vi "Create Group Buffers.vi"(8 "error in (no error)":errorcluster, 10 "Framework Configuration":refnum<class "Framework Configuration.lvclass">, 11 "VeriStand DSF in":refnum<class "VeriStand DSF.lvclass">) -> (0 "error out":errorcluster, 2 "Group Buffers":refnum<class "Buffers.lvclass">[](array[class]), 3 "VeriStand DSF out":refnum<class "VeriStand DSF.lvclass">)   [LabVIEW 2017, in "DSF Engine.lvlib" / "VeriStand DSF.lvclass"]
uses:
  VeriStand DSF.lvclass
  DSF Core.lvlibp/Classes/Buffers/Buffers.lvclass
  DSF Core.lvlibp/Classes/Configuration/Core/Framework/Framework Configuration.lvclass
  VeriStand DSF.lvclass/VeriStand DSF.ctl
  <vilib>/NI Veristand/Custom Device API/Data Access Type.ctl
  DSF Core.lvlibp/Typedefs/DSF Direction.ctl
  Shared/Data Channel Page GUID.vi
  DSF Core.lvlibp/Classes/Configuration/Core/Group/Group Configuration.lvclass
  Shared/DSF Shared.lvlib
  <vilib>/NI Veristand/Custom Device API/Custom Device API.lvlib
  DSF Core.lvlibp
  DSF Core.lvlibp/Classes/Configuration/Core/Transfer/Transfer Configuration.lvclass
  DSF Core.lvlibp/Classes/Configuration/Core/Thread/Thread Configuration.lvclass
  DSF Core.lvlibp/Classes/Configuration/Core/Plugin/Plugin Configuration.lvclass
  DSF Core.lvlibp/Classes/Buffer/Buffer.lvclass
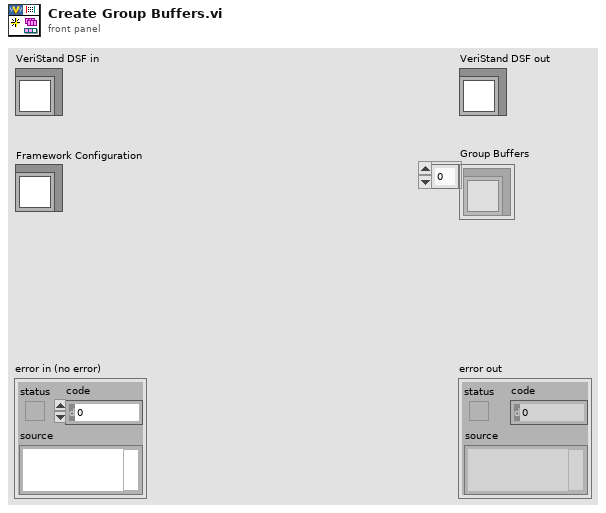
[diagram p1: front panel]
types:
  T1 = typedef "Custom Device API.lvlib/Custom Device Item Ref.ctl" = u64
  T2 = typedef "Custom Device API.lvlib/Data Access Type.ctl" = enum16{"Read", "Write"}
  T3 = typedef "DSF Core.lvlibp/DSF Direction.ctl" = enum8{"Tx", "Rx"}
  T4 = typedef "DSF Core.lvlibp/Group Configuration.lvclass/Core Group Configuration.ctl" = cluster{"name":string, "direction":T3, "cycle timing":T5, "timeout behavior":T6, "enable conversion":bool}
  T5 = typedef "DSF Core.lvlibp/DSF Timing Info.ctl" = cluster{"priority":u64, "decimation":u64, "offset":u64}
  T6 = typedef "DSF Core.lvlibp/DSF Timeout Behavior.ctl" = enum8{"Increment Late Count", "Throw Error"}
  T7 = typedef "DSF Core.lvlibp/Transfer Configuration.lvclass/Channel Configuration.ctl" = cluster{"configuration":T8, "component settings":T10[]}
  T8 = typedef "DSF Core.lvlibp/Channel Configuration.lvclass/Core Channel Configuration.ctl" = cluster{"name":string, "units":string, "engine data type":T9, "string data type":T9, "string offset":u64}
  T9 = typedef "DSF Core.lvlibp/DSF Data Type.ctl" = enum8{"Bool", "SGL", "DBL", "I8", "I16", "I32", "I64", "U8", "U16", "U32", "U64"}
  T10 = typedef "DSF Core.lvlibp/DSF Settings Info.ctl" = cluster{"component":string, "values":cluster{"key":string, "value":string}[]}
  T11 = typedef "Custom Device API.lvlib/Data Reference.ctl" = i32
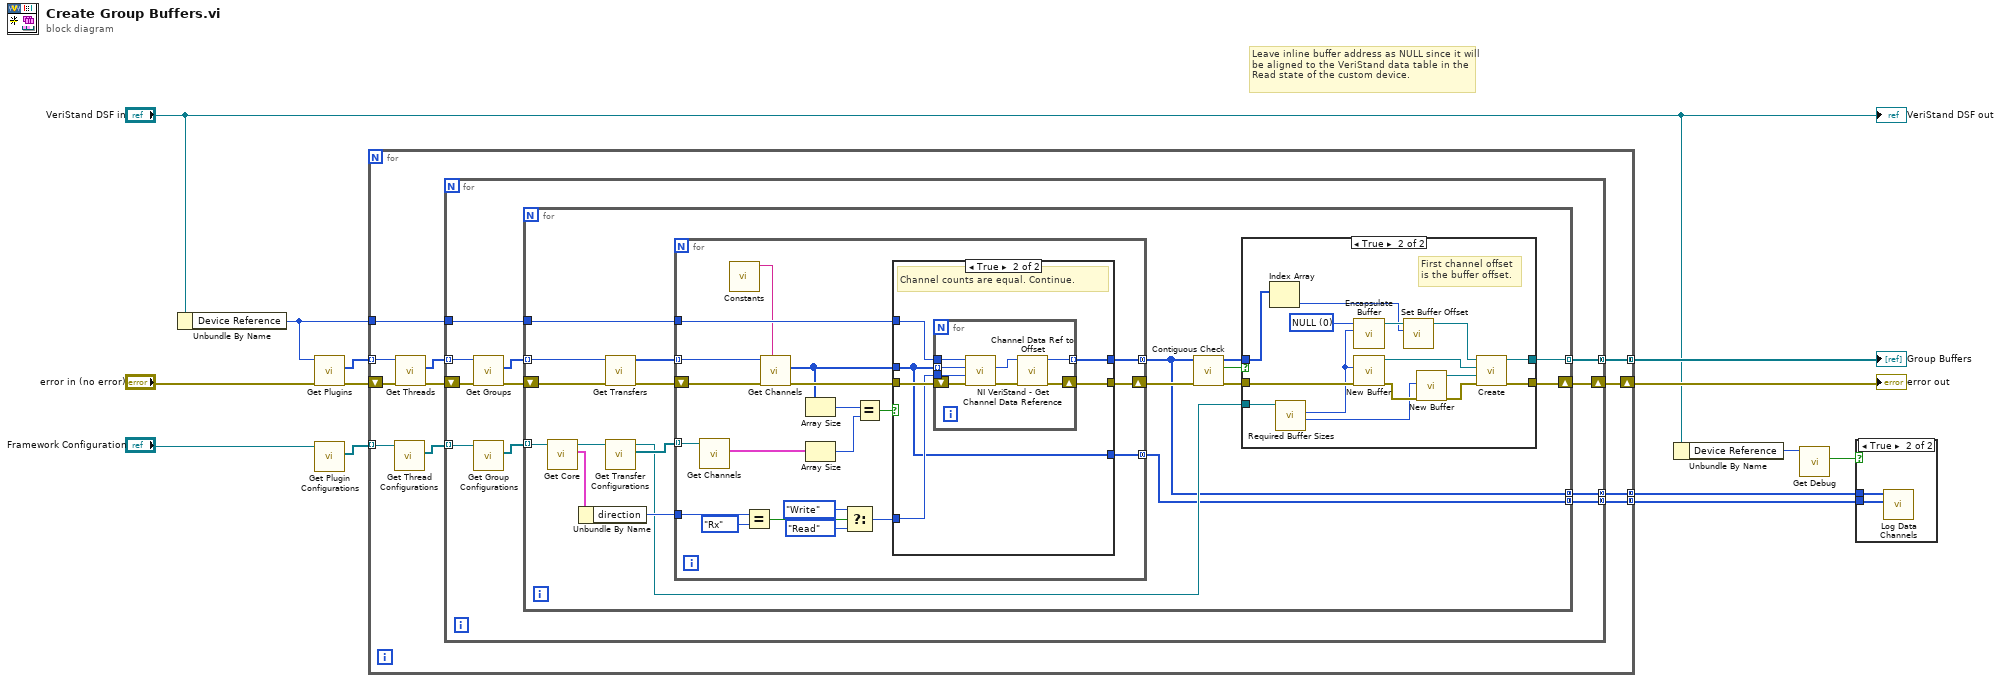
[diagram p0: block diagram]
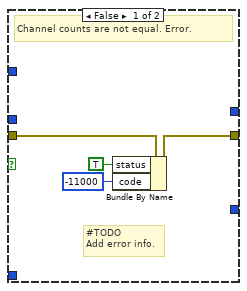
[diagram p2: hidden frame]
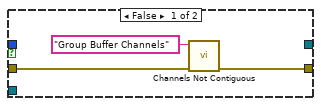
[diagram p3: hidden frame]
diagram:
  # "Leave inline buffer address as NULL since it will be aligned to the VeriStand data table in the Read state of the custom device."
  n1 = Unbundle By Name("VeriStand DSF in") -> ("Device Reference"=w8:T1)
  n2 = call "Get Plugins.vi"("error in (no error)"="error in (no error)", "Item Ref in"=w8) -> ("error out"=w13:errorcluster, "Plugin refs"=w12:T1[])  [unwired: 7 in, 1 out]
  n3 = call "Get Plugin Configurations.vi"("Framework Configuration in"="Framework Configuration") -> ("Plugin Configurations"=w11:refnum<class "Plugin Configuration.lvclass">[])  [unwired: 8 in, 2 out]
  n4 = for {
    tunnel: w12 -> [w21] mode=indexing
    tunnel: w8 -> [w23]
    tunnel: w11 -> [w18] mode=indexing
    shift-right: [w24] -> w2
    shift-left: w13 -> [w22]
    tunnel: [w16] -> w9 mode=concatenating
    tunnel: [w15] -> w4 mode=concatenating
    tunnel: [w14] -> w5 mode=concatenating
    n5 = call "Get Thread Configurations.vi"("Plugin Configuration in"=w18) -> ("Thread Configurations"=w17:refnum<class "Thread Configuration.lvclass">[])  [unwired: 8 in, 2 out]
    n6 = call "Get Threads.vi"("error in (no error)"=w22, "Item Ref in"=w21) -> ("error out"=w20:errorcluster, "Plugin refs"=w19:T1[])  [unwired: 7 in, 1 out]
    n7 = for {
      tunnel: w19 -> [w32] mode=indexing
      tunnel: w17 -> [w29] mode=indexing
      tunnel: w23 -> [w35]
      shift-right: [w34] -> w24
      shift-left: w20 -> [w33]
      tunnel: [w27] -> w16 mode=concatenating
      tunnel: [w26] -> w15 mode=concatenating
      tunnel: [w25] -> w14 mode=concatenating
      n8 = call "Get Groups.vi"("error in (no error)"=w33, "Plugin Ref in"=w32) -> ("error out"=w31:errorcluster, "Group refs"=w30:T1[])  [unwired: 7 in, 1 out]
      n9 = call "Get Group Configurations.vi"("Thread Configuration in"=w29) -> ("Group Configurations"=w28:refnum<class "Group Configuration.lvclass">[])  [unwired: 8 in, 2 out]
      n10 = for {
        tunnel: w28 -> [w40] mode=indexing
        tunnel: w30 -> [w53] mode=indexing
        tunnel: w35 -> [w39]
        shift-right: [w42] -> w34
        shift-left: w31 -> [w54]
        tunnel: [w41] -> w27 mode=indexing
        tunnel: [w37] -> w26 mode=concatenating
        tunnel: [w36] -> w25 mode=concatenating
        n11 = call "Get Core.vi"("Group Configuration in"=w40) -> ("core"=w47:T4, "Group Configuration out"=w50:refnum<class "Group Configuration.lvclass">)  [unwired: 8 in, 1 out]
        n12 = Unbundle By Name(w47) -> ("direction"=w48:T3)
        n13 = call "Get Transfers.vi"("error in (no error)"=w54, "Group Ref in"=w53) -> ("error out"=w52:errorcluster, "Transfer refs"=w51:T1[])  [unwired: 7 in, 1 out]
        n14 = call "Get Transfer Configurations.vi"("Group Configuration in"=w50) -> ("Transfer Configurations"=w49:refnum<class "Transfer Configuration.lvclass">[], "Group Configuration out"=w38:refnum<class "Group Configuration.lvclass">)  [unwired: 8 in, 1 out]
        n15 = for {
          tunnel: w49 -> [w58] mode=indexing
          tunnel: w51 -> [w65] mode=indexing
          tunnel: w39 -> [w69]
          shift-right: [w67] -> w46
          shift-left: w52 -> [w59]
          tunnel: [w66] -> w36 mode=concatenating
          tunnel: [w62] -> w37 mode=concatenating
          tunnel: w48 -> [w60]
          n16 = call "Get Channels.vi"("Transfer Configuration in"=w58) -> ("channels"=w57:T7[])  [unwired: 8 in, 2 out]
          n17 = call-poly "Constants.vi"() -> ("Status GUID"=w61:string)  [unwired: 11 in]
          n18 = Equal?(x=w60, y=DSF_Direction."Rx") -> (x = y?=w73:bool)
          n19 = call "Get Channels.vi"("GUID (Default Channel)"=w61, "error in (no error)"=w59, "Item Ref in"=w65) -> ("error out"=w64:errorcluster, "Channels refs"=w63:T1[])  [unwired: 6 in, 1 out]
          n20 = Array Size(array=w63) -> (size(s)=w55:i32)
          n21 = Array Size(array=w57) -> (size(s)=w56:i32)
          n22 = Select(t=Data_Access_Type."Write" ("Access"), s=w73, f=Data_Access_Type."Read") -> (s? t:f=w68:T2)
          n23 = Equal?(x=w55, y=w56) -> (x = y?=w70:bool)
          n24 = case shown="True" w70 {
            tunnel: w63 -> [_ w79]
            tunnel: w69 -> [_ w83]
            tunnel: w68 -> [_ w82]
            tunnel: w64 -> [w78 w84]
            tunnel: [w77 w80] -> w67
            tunnel: [_ w81] -> w66
            tunnel: [_ w79] -> w62
            frame False {
              # "#TODO\nAdd error info."
              # "Channel counts are not equal. Error."
              n25 = Bundle By Name(cluster=w78, "status"=TRUE, "code"=-11000) -> (w77:errorcluster)
            }
            frame True {
              # "Channel counts are equal. Continue."
              n26 = for {
                tunnel: w83 -> [w91]
                tunnel: w82 -> [w90]
                tunnel: w79 -> [w89] mode=indexing
                tunnel: [w85] -> w81 mode=indexing
                shift-right: [w86] -> w80
                shift-left: w84 -> [w92]
                n27 = call <vilib>:"NI VeriStand - Get Channel Data Reference.vi"("error in (no error)"=w92, "Access"=w90, "Channel Ref in"=w89, "Device Ref in"=w91) -> ("error out"=w88:errorcluster, "Channel Data Reference"=w87:T11)  [unwired: 5 in, 1 out]
                n28 = call "Channel Data Ref to Offset.vi"("error in (no error)"=w88, "Channel Data Reference"=w87) -> ("error out"=w86:errorcluster, "channel offset"=w85:u64)  [unwired: 8 in]
              }
            }
          }
        }
        n29 = call "Contiguous Check.vi"("error in (no error)"=w46, "channel offsets in"=w36) -> ("error out"=w45:errorcluster, "contiguous?"=w44:bool, "channel offsets out"=w43:u64[])  [unwired: 7 in]
        n30 = case shown="True" w44 {
          tunnel: [w95 w110] -> w42
          tunnel: w45 -> [w94 w103]
          tunnel: w43 -> [_ w107]
          tunnel: [_ w109] -> w41
          tunnel: w38 -> [_ w105]
          frame False {
            n31 = call "Channels Not Contiguous.vi"("error in (no error)"=w94, "name"="Group Buffer Channels") -> ("error out"=w95:errorcluster)  [unwired: 9 in]
          }
          frame True {
            w99 = u64 0 items=["NULL"]
            # "First channel offset is the buffer offset."
            n32 = Index Array(array=w107) -> (element=w106:u64)  [unwired: 1 in]
            n33 = call-dynamic "Required Buffer Sizes.vi"("Group Configuration in"=w105) -> ("string size"=w96:u64, "engine size"=w97:u64)  [unwired: 7 in, 2 out]
            n34 = call "Encapsulate Buffer.vi"("buffer size"=w97, "buffer address"=w99) -> ("Buffer"=w108:refnum<class "Buffer.lvclass">)  [unwired: 8 in, 1 out]
            n35 = call "New Buffer.vi"("error in (no error)"=w103, "buffer size"=w97) -> ("error out"=w98:errorcluster, "Buffer out"=w102:refnum<class "Buffer.lvclass">)  [unwired: 8 in]
            n36 = call "Set Buffer Offset.vi"("buffer offset"=w106, "Buffer in"=w108) -> ("Buffer out"=w104:refnum<class "Buffer.lvclass">)  [unwired: 9 in]
            n37 = call "New Buffer.vi"("error in (no error)"=w98, "buffer size"=w96) -> ("error out"=w100:errorcluster, "Buffer out"=w101:refnum<class "Buffer.lvclass">)  [unwired: 8 in]
            n38 = call "Create.vi"("error in (no error)"=w100, "String Buffer (null)"=w101, "Async Buffer (null)"=w102, "Inline Buffer (null)"=w104) -> ("error out"=w110:errorcluster, "Buffers out"=w109:refnum<class "Buffers.lvclass">)  [unwired: 6 in]
          }
        }
      }
    }
  }
  "error out" <- w2
  "Group Buffers" <- w9
  n39 = Unbundle By Name("VeriStand DSF in") -> ("Device Reference"=w6:T1)
  n40 = call "Get Debug.vi"("Item Ref in"=w6) -> ("debug"=w3:bool)  [unwired: 8 in, 2 out]
  n41 = case shown="True" w3 {
    tunnel: w4 -> [_ w112]
    tunnel: w5 -> [_ w111]
    frame False {
    }
    frame True {
      n42 = call "Log Data Channels.vi"("data channels refs"=w112, "data channel offsets"=w111) -> ()  [unwired: 10 in]
    }
  }
  "VeriStand DSF out" <- "VeriStand DSF in"
